vi "New Message.vi"(8 "error in (no error)":errorcluster, 10 "TcpPayload":T1, 11 "RemoteMessaging in":refnum<class "RemoteMessaging.lvclass">) -> (0 "error out":errorcluster, 3 "RemoteMessaging out":refnum<class "RemoteMessaging.lvclass">)   [LabVIEW 2020, in "Volatus.lvlib" / "RemoteMessaging.lvclass"]
uses:
  RemoteMessaging.lvclass
  C:/dev/lv20CE/relink/lv-volatus/Volatus/Task/Task.lvclass
  lv-vecto/Vecto/proto/TcpPayload/Data.ctl
  RemoteMessaging.lvclass/RemoteMessaging.ctl
  Event Level.ctl
  Task/Task.lvclass/Task.ctl
  VolatusAPI/VolatusAPI.lvclass/VolatusAPI.ctl
  Event API/EventAPI.lvclass/EventAPI.ctl
  EventHandler Messages/Handle Event Msg/Handle Event Msg.lvclass/Handle Event Msg.ctl
  <vilib>/ActorFramework/Message Enqueuer/Message Enqueuer.lvclass/Message Enqueuer.ctl
  EventHandler Messages/Handle Event Msg/Send Handle Event.vi
  <vilib>/ActorFramework/Message Enqueuer/Enqueue.vi
  EventHandler Messages/Handle Event Msg/Handle Event Msg.lvclass
  C:/Program Files (x86)/National Instruments/LabVIEW 2020/vi.lib/ActorFramework/Message/Message.lvclass
  <vilib>/ActorFramework/Message Priority Queue/Priority Enqueue.vi
  Task/Task.lvclass
  Volatus.lvlib
  RemoteCommandable Messages/Handle Message Msg/Handle Message Msg.lvclass
  lv-vecto/Vecto/proto/TcpPayload/TcpPayload.lvlib
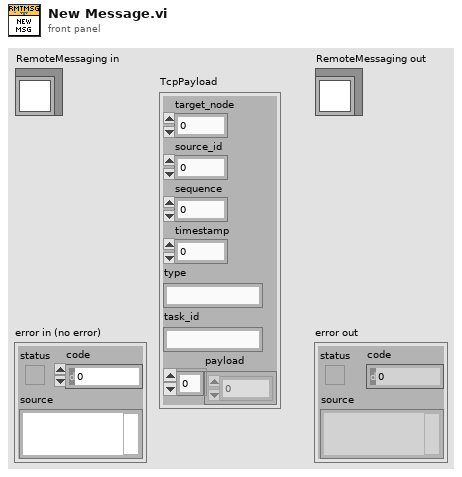
[diagram p1: front panel]
types:
  T1 = typedef "TcpPayload.lvlib/Data.ctl" = cluster{"target_node":u32, "source_id":u32, "sequence":u32, "timestamp":u64, "type":string, "task_id":string, "payload":u8[]}
  T2 = map{string, refnum<class "Message Enqueuer.lvclass">[]}
  T3 = typedef "Volatus.lvlib/Event Level.ctl" = enum16{"Debug", "Info", "Warning", "Error"}
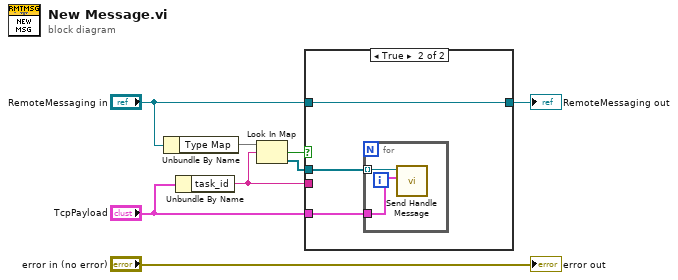
[diagram p0: block diagram]
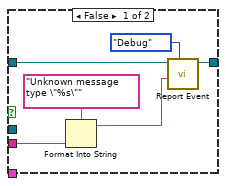
[diagram p2: hidden frame]
diagram:
  n1 = Unbundle By Name("RemoteMessaging in") -> ("Type Map"=w7:T2)
  n2 = Unbundle By Name("TcpPayload") -> ("task_id"=w3:string)
  n3 = Look In Map(map=w7, key=w3) -> (key not found?=w6:bool, value=w5:refnum<class "Message Enqueuer.lvclass">[])  [unwired: 1 in]
  n4 = case shown="True" w6 {
    tunnel: w5 -> [_ w17]
    tunnel: "RemoteMessaging in" -> [w14 w15]
    tunnel: w3 -> [w12 _]
    tunnel: "TcpPayload" -> [_ w16]
    tunnel: [w9 w15] -> w1
    frame False {
      n5 = Format Into String(format string="Unknown message type \"%s\"", w12) -> (resulting string=w10:string)  [unwired: 2 in, 1 out]
      n6 = call "Report Event.vi"("Level (Info)"=Event_Level."Debug", "Message"=w10, "Task in"=w14) -> ("Task out"=w9:refnum<class "RemoteMessaging.lvclass">)  [unwired: 7 in, 1 out]
    }
    frame True {
      n7 = for {
        tunnel: w17 -> [w19] mode=indexing
        tunnel: w16 -> [w18]
        n8 = call "Send Handle Message.vi"("TcpPayload"=w18, "Message Enqueuer"=w19) -> ()  [unwired: 8 in, 2 out]
      }
    }
  }
  "RemoteMessaging out" <- w1
  "error out" <- "error in (no error)"
